vi "EncoderActuallDistance.vi"(11 "Wheel Diameter":dbl) -> (3 "DistancePerCount":dbl)   [LabVIEW 2015]
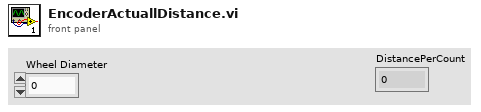
[diagram p1: front panel]
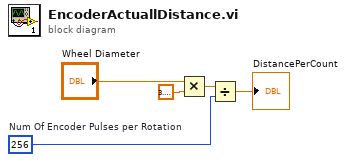
[diagram p0: block diagram]
diagram:
  w3 = 256  # Num Of Encoder Pulses per Rotation
  n1 = Multiply(x="Wheel Diameter", y=3.141592653589793) -> (x*y=w4:dbl)
  n2 = Divide(x=w4, y=w3) -> (x/y=→"DistancePerCount":dbl)
